vi "Komunikat_OK.vi"(1 "String 2":string) -> (0 "OUT":bool)   [LabVIEW 2019]
panel:
  in  "OK":bool
  out "String":string
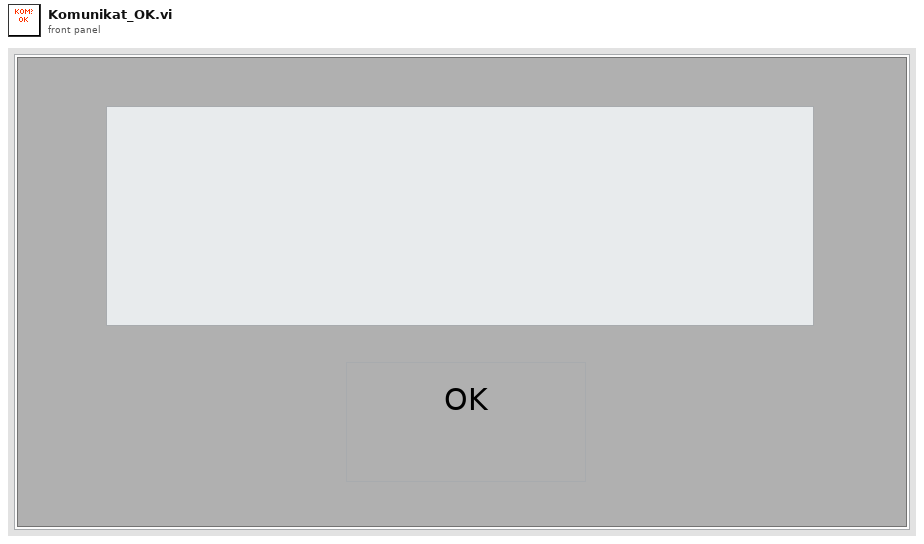
[diagram p1: front panel]
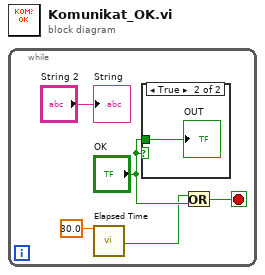
[diagram p0: block diagram]
diagram:
  n1 = while {
    stop <- w3 stop-if-true
    n2 = call "Elapsed Time"("Time Target (s)"=30.0) -> ("Time has Elapsed"=w1:bool)  [unwired: 11 in, 7 out]
    n3 = case shown="True" "OK" {
      tunnel: "OK" -> [_ w6]
      frame False {
      }
      frame True {
        "OUT" <- w6
      }
    }
    n4 = Or(x=w1, y="OK") -> (x .or. y?=w3:bool)
    "String" <- "String 2"
  }
